vi "Find Corners in sub.vi"(3 "Start point":cluster{"X":dbl, "Y":dbl}, 4 "Sub Matrix\n(Object edge)":T1) -> (1 "Corners":cluster{"X":dbl, "Y":dbl}[](array[cluster]))   [LabVIEW 2009]
uses:
  <vilib>/Analysis/Matrix/Datatypes/RealMatrix.ctl
  <vilib>/Analysis/Matrix/NI_Matrix.lvlib
panel:
  in  "Corner candidate":cluster{"X":dbl, "Y":dbl}
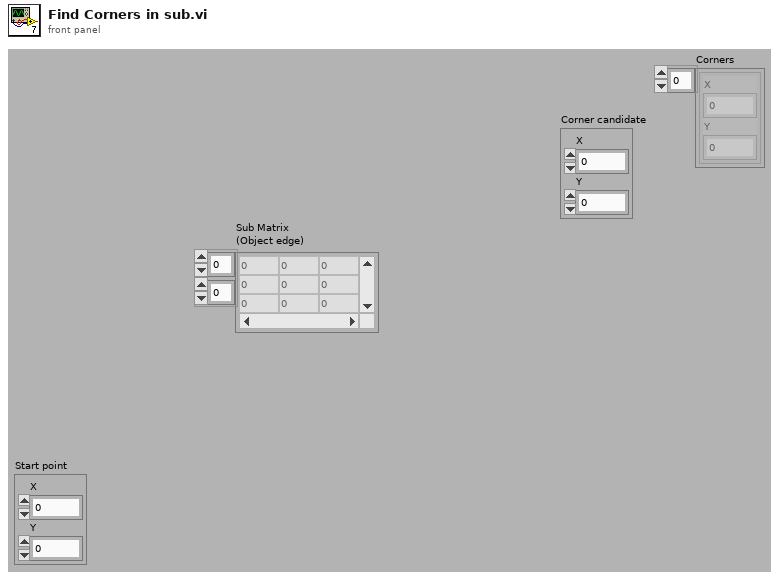
[diagram p1: front panel]
types:
  T1 = typedef "NI_Matrix.lvlib/RealMatrix.ctl" = dbl[][]
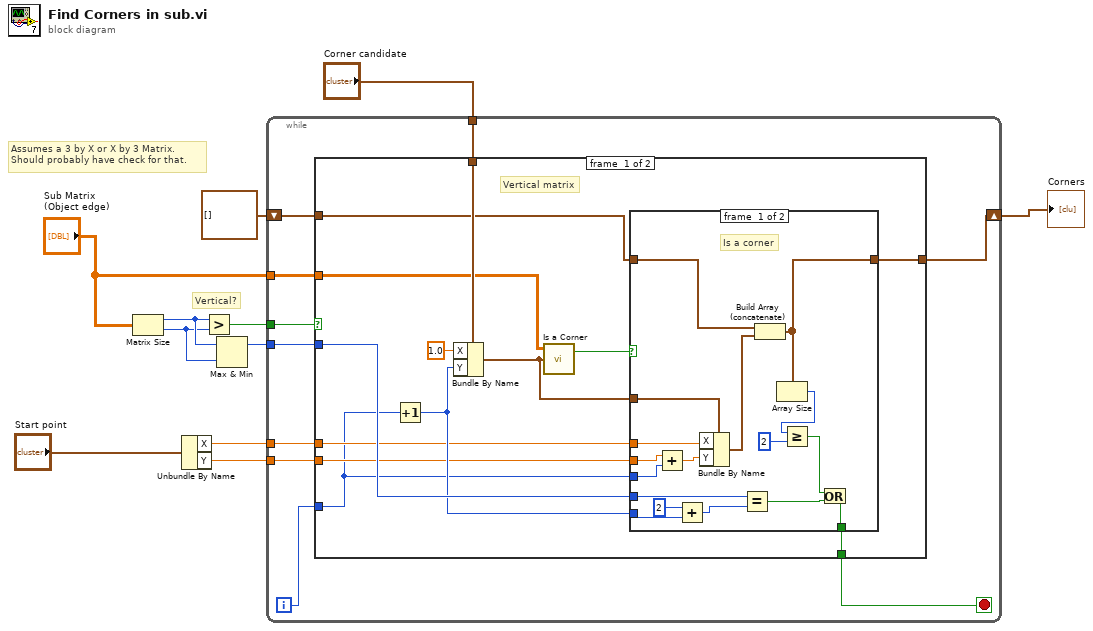
[diagram p0: block diagram]
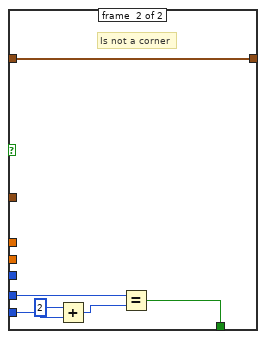
[diagram p2: hidden frame]
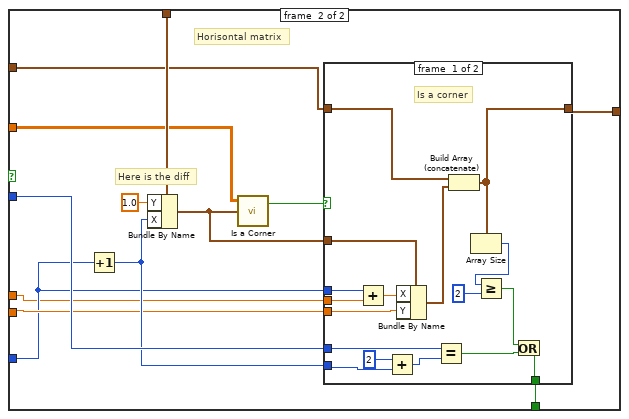
[diagram p3: hidden frame]
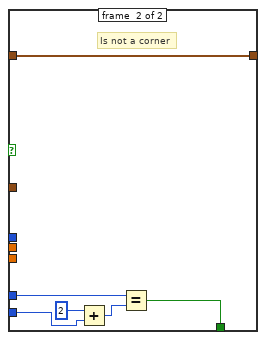
[diagram p4: hidden frame]
diagram:
  # "Assumes a 3 by X or X by 3 Matrix.\nShould probably have check for that."
  # "Vertical?"
  n1 = Matrix Size(0:"Sub Matrix\n(Object edge)") -> (1:w10:i32, 2:w9:i32)
  n2 = Unbundle By Name("Start point") -> ("X"=w3:dbl, "Y"=w2:dbl)
  n3 = Greater?(x=w10, y=w9) -> (0:w11:bool)
  n4 = Max & Min(x=w10, y=w9) -> (max(x,y)=w8:i32)  [unwired: 1 out]
  n5 = while {
    tunnel: w11 -> [w21]
    tunnel: w8 -> [w20]
    tunnel: "Corner candidate" -> [w19]
    tunnel: "Sub Matrix\n(Object edge)" -> [w18]
    shift-right: [w15] -> w5
    shift-left: cluster{"X":dbl, "Y":dbl}[] [] -> [w14]
    tunnel: w3 -> [w13]
    tunnel: w2 -> [w12]
    i -> [w17]
    stop <- w16 stop-if-true
    n6 = case shown="False" w21 {
      tunnel: w20 -> [w30 w66]
      tunnel: w19 -> [w34 w70]
      tunnel: w18 -> [w32 w68]
      tunnel: w17 -> [w22 w59]
      tunnel: [w29 w65] -> w16
      tunnel: [w27 w63] -> w15
      tunnel: w14 -> [w26 w62]
      tunnel: w13 -> [w24 w58]
      tunnel: w12 -> [w23 w60]
      frame #0 {
        # "Vertical matrix"
        n7 = Increment(x=w22) -> (x+1=w28:i32)
        n8 = Bundle By Name(cluster=w34, "X"=1.0, "Y"=w28) -> (w25:cluster{"X":dbl, "Y":dbl})
        n9 = call "Is a Corner.vi"("Corner candidate"=w25, "Updated Map"=w32) -> ("Is a corner"=w31:bool)  [unwired: 2 in]
        n10 = case shown="True" w31 {
          tunnel: [w42 w52] -> w27
          tunnel: w28 -> [w44 w54]
          tunnel: w30 -> [w49 w57]
          tunnel: [w46 w56] -> w29
          tunnel: w25 -> [w40 _]
          tunnel: w26 -> [w41 w52]
          tunnel: w24 -> [w38 _]
          tunnel: w23 -> [w36 _]
          tunnel: w22 -> [w35 _]
          frame #0 {
            # "Is a corner"
            n11 = Add(x=w36, y=w35) -> (x+y=w37:dbl)
            n12 = Add(x=2, y=w44) -> (x+y=w45:i32)
            n13 = Bundle By Name(cluster=w40, "X"=w38, "Y"=w37) -> (w39:cluster{"X":dbl, "Y":dbl})
            n14 = Equal?(x=w49, y=w45) -> (x = y?=w47:bool)
            n15 = Build Array (concatenate)(w41, w39) -> (w42:cluster{"X":dbl, "Y":dbl}[])
            n16 = Array Size(array=w42) -> (size(s)=w51:i32)
            n17 = Greater Or Equal?(x=w51, y=2) -> (x >= y?=w48:bool)
            n18 = Or(x=w48, y=w47) -> (x .or. y?=w46:bool)
          }
          frame #1 {
            # "Is not a corner"
            n19 = Add(x=2, y=w54) -> (x+y=w55:i32)
            n20 = Equal?(x=w57, y=w55) -> (x = y?=w56:bool)
          }
        }
      }
      frame #1 {
        # "Here is the diff"
        # "Horisontal matrix"
        n21 = Increment(x=w59) -> (x+1=w64:i32)
        n22 = Bundle By Name(cluster=w70, "Y"=1.0 ("X"), "X"=w64) -> (w61:cluster{"X":dbl, "Y":dbl})
        n23 = call "Is a Corner.vi"("Corner candidate"=w61, "Updated Map"=w68) -> ("Is a corner"=w67:bool)  [unwired: 2 in]
        n24 = case shown="True" w67 {
          tunnel: w64 -> [w80 w89]
          tunnel: w66 -> [w85 w93]
          tunnel: [w82 w92] -> w65
          tunnel: w61 -> [w76 _]
          tunnel: [w78 w88] -> w63
          tunnel: w62 -> [w77 w88]
          tunnel: w60 -> [w73 _]
          tunnel: w59 -> [w72 _]
          tunnel: w58 -> [w71 _]
          frame #0 {
            # "Is a corner"
            n25 = Add(x=w72, y=w71) -> (x+y=w74:dbl)
            n26 = Add(x=2, y=w80) -> (x+y=w81:i32)
            n27 = Bundle By Name(cluster=w76, "X"=w74, "Y"=w73) -> (w75:cluster{"X":dbl, "Y":dbl})
            n28 = Equal?(x=w85, y=w81) -> (x = y?=w83:bool)
            n29 = Build Array (concatenate)(w77, w75) -> (w78:cluster{"X":dbl, "Y":dbl}[])
            n30 = Array Size(array=w78) -> (size(s)=w87:i32)
            n31 = Greater Or Equal?(x=w87, y=2) -> (x >= y?=w84:bool)
            n32 = Or(x=w84, y=w83) -> (x .or. y?=w82:bool)
          }
          frame #1 {
            # "Is not a corner"
            n33 = Add(x=2, y=w89) -> (x+y=w90:i32)
            n34 = Equal?(x=w93, y=w90) -> (x = y?=w92:bool)
          }
        }
      }
    }
  }
  "Corners" <- w5
